vi "Get Module Execution Status by ref.vi"(6 "Modules Tree ref":refnum<vi>, 10 "Modules Types":T1[](array[typedef]), 11 "Library":refnum<vi>[](array[refnum])) -> (0 "error out":errorcluster)   [LabVIEW 2019, in "Panther Dashboard.lvlib"]
doc: "This VI checks the Main.vi State of the selected DQMH Module"
uses:
  Panther Dashboard.lvlib
  Module type--enum.ctl
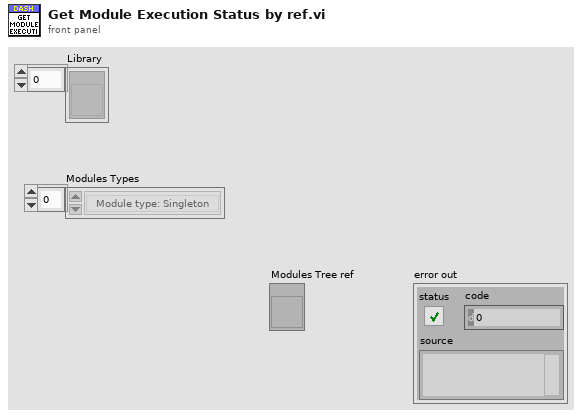
[diagram p1: front panel]
types:
  T1 = typedef "Panther Dashboard.lvlib/Module type--enum.ctl" = enum16{"Module type: Singleton", "Module type: Cloneable"}
  T2 = typedef "imagedata.ctl" = cluster{"image type":i32, "image depth":i32, "image":u8[], "mask":u8[], "colors":u32[], "Rectangle":cluster{"left":i16, "top":i16, "right":i16, "bottom":i16}}
  T3 = enum32{"Bad", "Idle", "Run top level", "Running"}
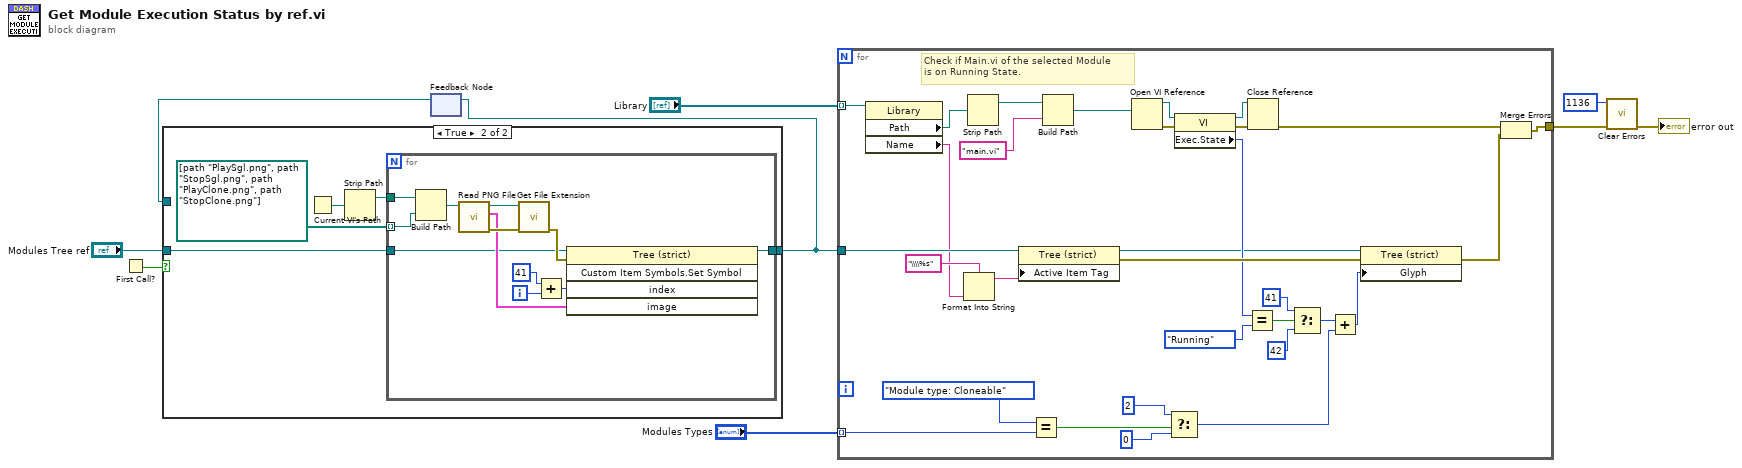
[diagram p0: block diagram]
diagram:
  n1 = First Call?() -> (First Call?: T/F=w5:bool)
  n2 = feedback #1() -> (w2:refnum<vi>)  [unwired: 1 in]
  n3 = case shown="True" w5 {
    tunnel: [w10 w13] -> w3
    tunnel: "Modules Tree ref" -> [_ w11]
    tunnel: w2 -> [w10 _]
    frame False {
    }
    frame True {
      n4 = Current VI's Path() -> (path=w15:path)
      n5 = Strip Path(path=w15) -> (stripped path=w12:path)  [unwired: 1 out]
      n6 = for {
        tunnel: w12 -> [w24]
        tunnel: path[] [path "PlaySgl.png", path "StopSgl.png", path "PlayClone.png", path "StopClone.png"] ("name or relative path") -> [w23] mode=indexing
        tunnel: w11 -> [w17]
        tunnel: [w16] -> w13
        i -> [w20]
        n7 = Build Path(base path=w24, name or relative path=w23) -> (appended path=w22:path)
        n8 = call <vilib>:"Read PNG File.vi"("path to PNG file"=w22) -> ("error out"=w27:errorcluster, "image data"=w19:T2, "path"=w25:path)  [unwired: 8 in]
        n9 = call <vilib>:"Get File Extension.vi"("error in (no error)"=w27, "file"=w25) -> ("error out"=w26:errorcluster)  [unwired: 5 in, 4 out]
        n10 = Add(x=41 ("Index"), y=w20) -> (x+y=w18:i32)
        n11 = invoke on="Invoke Node" class="Tree (strict)" method="Custom Item Symbols.Set Symbol"(reference=w17, error in=w26, "index"=w18, "image"=w19) -> (reference out=w16:refnum<vi>)  [unwired: 1 in, 4 out]
      }
    }
  }
  n12 = feedback-in #1(w3) -> ()
  n13 = for {
    tunnel: [w54] -> w9
    tunnel: "Library" -> [w44] mode=indexing
    tunnel: w3 -> [w43]
    tunnel: "Modules Types" -> [w33] mode=indexing
    # "Check if Main.vi of the selected Module\nis on Running State."
    n14 = property class="Library"(reference=w44) -> ("Path"=w52:path, "Name"=w35:string)  [unwired: 1 in, 2 out]
    n15 = Format Into String(format string="\\\\%s", w35) -> (resulting string=w42:string)  [unwired: 2 in, 1 out]
    n16 = Strip Path(path=w52) -> (stripped path=w51:path)  [unwired: 1 out]
    n17 = property class="Tree (strict)"(reference=w43, "Active Item Tag"=w42) -> (reference out=w41:refnum<vi>, error out=w55:errorcluster)  [unwired: 1 in]
    n18 = Equal?(x=Module_type--enum."Module type: Cloneable", y=w33) -> (x = y?=w31:bool)
    n19 = Build Path(base path=w51, name or relative path="main.vi" ("string")) -> (appended path=w49:path)
    n20 = Open VI Reference(vi path=w49) -> (vi reference=w48:refnum<vi>, error out=w56:errorcluster)  [unwired: 5 in]
    n21 = Select(t=2, s=w31, f=0) -> (s? t:f=w28:i32)
    n22 = property class="VI"(reference=w48, error in=w56) -> (reference out=w45:refnum<vi>, error out=w57:errorcluster, "Exec.State"=w47:T3)
    n23 = Equal?(x=w47, y=T3."Running") -> (x = y?=w38:bool)
    n24 = Close Reference(reference=w45, error in (no error)=w57) -> (error out=w58:errorcluster)
    n25 = Select(t=41, s=w38, f=42) -> (s? t:f=w40:i32)
    n26 = Add(x=w40, y=w28) -> (x+y=w34:i32)
    n27 = property class="Tree (strict)"(reference=w41, error in=w55, "Glyph"=w34) -> (error out=w53:errorcluster)  [unwired: 1 out]
    n28 = Merge Errors(w58, w53) -> (w54:errorcluster)
  }
  n29 = call <vilib>:"Clear Errors.vi"("error in (no error)"=w9, "specific error code to clear (0: all)"=1136) -> ("error out"=→"error out":errorcluster)  [unwired: 4 in, 1 out]
